vi "WriteIni.vi"(1 "configuration file path":path) -> ()   [LabVIEW 2018]
uses:
  <vilib>/Utility/config.llb/Write Key (String).vi
  <vilib>/Utility/config.llb/Write Key (I32).vi
  <vilib>/Utility/config.llb/NI_LVConfig.lvlib
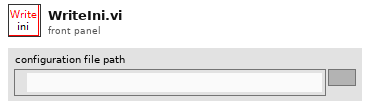
[diagram p1: front panel]
types:
  T1 = typedef "NI_LVConfig.lvlib/Config Data RefNum.ctl" = refnum<k1>
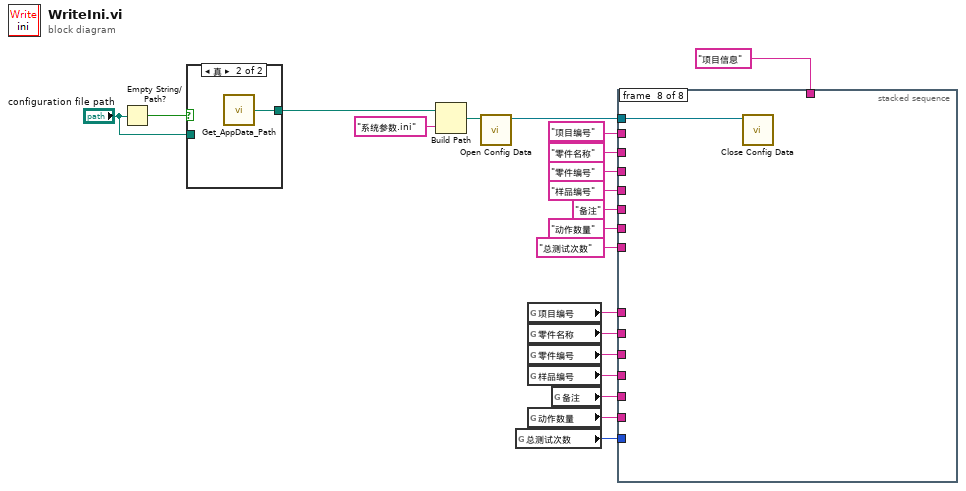
[diagram p0: block diagram]
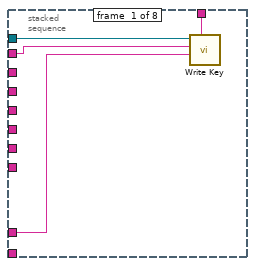
[diagram p3: hidden frame]
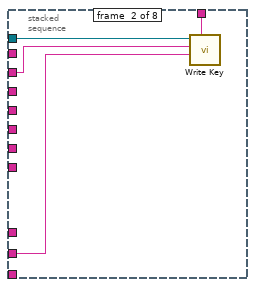
[diagram p4: hidden frame]
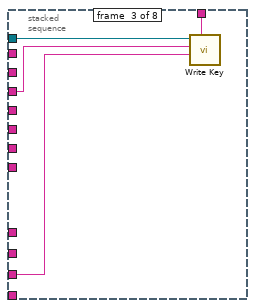
[diagram p5: hidden frame]
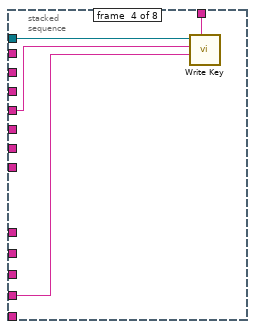
[diagram p6: hidden frame]
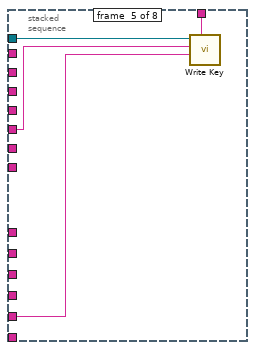
[diagram p7: hidden frame]
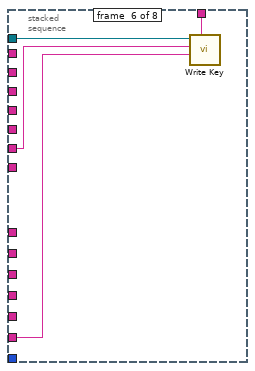
[diagram p8: hidden frame]
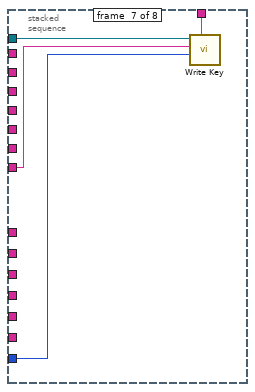
[diagram p9: hidden frame]
diagram:
  n1 = Empty String/Path?(string/path="configuration file path") -> (empty?=w3:bool)
  n2 = case shown="真" w3 {
    tunnel: [w22 w23] -> w2
    tunnel: "configuration file path" -> [w22 _]
    frame False {
    }
    frame True {
      n3 = call "Get_AppData_Path.vi"() -> ("path"=w23:path)  [unwired: 1 in]
    }
  }
  n4 = Build Path(base path=w2, name or relative path="系统参数.ini" ("名称或相对路径")) -> (appended path=w21:path)
  n5 = call <vilib>:"Open Config Data.vi"("configuration file path"=w21) -> ("refnum"=w20:T1)  [unwired: 8 in, 2 out]
  n6 = global read "全局 1.vi" "总测试次数"() -> (w4:i16)
  n7 = global read "全局 1.vi" "项目编号"() -> (w10:string)
  n8 = global read "全局 1.vi" "零件名称"() -> (w9:string)
  n9 = global read "全局 1.vi" "零件编号"() -> (w8:string)
  n10 = global read "全局 1.vi" "样品编号"() -> (w7:string)
  n11 = global read "全局 1.vi" "动作数量"() -> (w5:string)
  n12 = global read "全局 1.vi" "备注"() -> (w6:string)
  n13 = stacked-sequence {
    tunnel: w20 -> [w27 w31 w35 w39 w43 w47 w51 w52]
    tunnel: "项目编号" -> [w26 _ _ _ _ _ _ _]
    tunnel: "零件名称" -> [_ w30 _ _ _ _ _ _]
    tunnel: "零件编号" -> [_ _ w33 _ _ _ _ _]
    tunnel: "样品编号" -> [_ _ _ w37 _ _ _ _]
    tunnel: "备注" -> [_ _ _ _ w41 _ _ _]
    tunnel: "动作数量" -> [_ _ _ _ _ w45 _ _]
    tunnel: "总测试次数" -> [_ _ _ _ _ _ w49 _]
    tunnel: "项目信息" -> [w25 w29 w34 w38 w42 w46 w50 _]
    tunnel: w10 -> [w24 _ _ _ _ _ _ _]
    tunnel: w9 -> [_ w28 _ _ _ _ _ _]
    tunnel: w8 -> [_ _ w32 _ _ _ _ _]
    tunnel: w7 -> [_ _ _ w36 _ _ _ _]
    tunnel: w6 -> [_ _ _ _ w40 _ _ _]
    tunnel: w5 -> [_ _ _ _ _ w44 _ _]
    tunnel: w4 -> [_ _ _ _ _ _ w48 _]
    frame #0 {
      n14 = call-poly <vilib>:"Write Key.vi"("section"=w25, "value"=w24, "key"=w26, "refnum"=w27) -> ()  [unwired: 5 in, 3 out]
    }
    frame #1 {
      n15 = call-poly <vilib>:"Write Key.vi"("section"=w29, "value"=w28, "key"=w30, "refnum"=w31) -> ()  [unwired: 5 in, 3 out]
    }
    frame #2 {
      n16 = call-poly <vilib>:"Write Key.vi"("section"=w34, "value"=w32, "key"=w33, "refnum"=w35) -> ()  [unwired: 5 in, 3 out]
    }
    frame #3 {
      n17 = call-poly <vilib>:"Write Key.vi"("section"=w38, "value"=w36, "key"=w37, "refnum"=w39) -> ()  [unwired: 5 in, 3 out]
    }
    frame #4 {
      n18 = call-poly <vilib>:"Write Key.vi"("section"=w42, "value"=w40, "key"=w41, "refnum"=w43) -> ()  [unwired: 5 in, 3 out]
    }
    frame #5 {
      n19 = call-poly <vilib>:"Write Key.vi"("section"=w46, "value"=w44, "key"=w45, "refnum"=w47) -> ()  [unwired: 5 in, 3 out]
    }
    frame #6 {
      n20 = call-poly <vilib>:"Write Key.vi"("section"=w50, "value"=w48, "key"=w49, "refnum"=w51) -> ()  [unwired: 5 in, 3 out]
    }
    frame #7 {
      n21 = call <vilib>:"Close Config Data.vi"("refnum"=w52) -> ()  [unwired: 9 in, 2 out]
    }
  }
